vi "ConcatenateLabel.vi"(10 "Unit":string, 11 "Label in":string) -> (1 "Boolean":bool, 2 "Unit (dup)":string, 3 "Label out":string)   [LabVIEW 2017, in "XListGraph.lvlib" / "XListGraph.xctl"]
uses:
  XListGraph.xctl
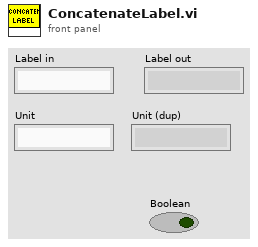
[diagram p1: front panel]
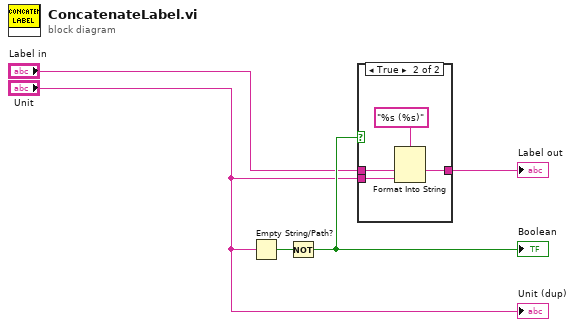
[diagram p0: block diagram]
diagram:
  n1 = Empty String/Path?(string/path="Unit") -> (empty?=w2:bool)
  n2 = Not(x=w2) -> (.not. x?=w5:bool)
  "Boolean" <- w5
  n3 = case shown="True" w5 {
    tunnel: "Label in" -> [w6 w9]
    tunnel: "Unit" -> [_ w8]
    tunnel: [w6 w7] -> w4
    frame False {
    }
    frame True {
      n4 = Format Into String(format string="%s (%s)", w9, w8) -> (resulting string=w7:string)  [unwired: 2 in, 1 out]
    }
  }
  "Label out" <- w4
  "Unit (dup)" <- "Unit"
